vi "SaveText.vi"(7 "action":string="Save", 8 "error in":errorcluster, 10 "data in":sgl, 11 "file path (use dialog)":path) -> (0 "error out":errorcluster)   [LabVIEW 2018]
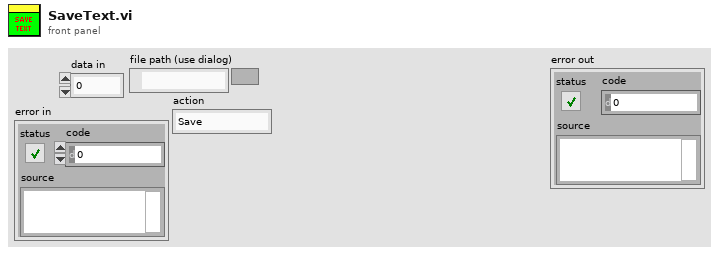
[diagram p1: front panel]
types:
  T1 = enum16{"open", "replace", "create", "open or create", "replace or create", "replace or create with confirmation"}
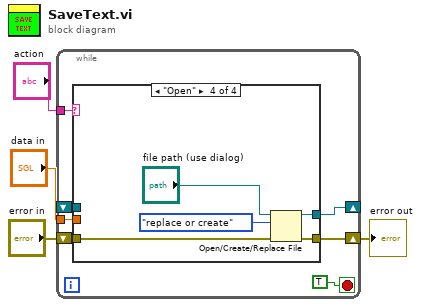
[diagram p0: block diagram]
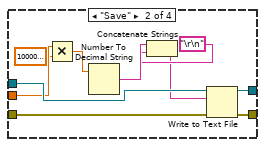
[diagram p3: hidden frame]
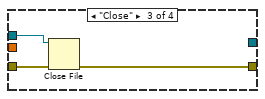
[diagram p4: hidden frame]
diagram:
  n1 = while {
    tunnel: "action" -> [w10]
    tunnel: "data in" -> [w9]
    shift-right: [w7] -> w1
    shift-left: "error in" -> [w8]
    shift-right: [w6] -> _
    shift-left: _ -> [w5]
    stop <- TRUE stop-if-true
    n2 = case shown="\"Open\"" w10 {
      tunnel: w9 -> [_ w16 _ _]
      tunnel: w8 -> [w13 w23 w26 w29]
      tunnel: [w13 w22 w24 w27] -> w7
      tunnel: [w12 w21 _ w31] -> w6
      tunnel: w5 -> [w12 w20 w25 _]
      frame "False", Default {
      }
      frame "Save" {
        n3 = Multiply(x=w16, y=sgl 1000000.0) -> (x*y=w14:sgl)
        n4 = Number To Decimal String(number=w14) -> (decimal integer string=w19:string)  [unwired: 1 in]
        n5 = Concatenate Strings(w19, "\r\n") -> (w17:string)
        n6 = Write to Text File(file (use dialog)=w20, text=w17, error in=w23) -> (refnum out=w21:refnum<file>, error out=w22:errorcluster)  [unwired: 1 in, 1 out]
      }
      frame "Close" {
        n7 = Close File(refnum=w25, error in=w26) -> (error out=w24:errorcluster)  [unwired: 1 out]
      }
      frame "Open" {
        n8 = Open/Create/Replace File(file path (use dialog)="file path (use dialog)", error in=w29, operation (0:open)=T1."replace or create") -> (refnum out=w31:refnum<file>, error out=w27:errorcluster)  [unwired: 3 in, 1 out]
      }
    }
  }
  "error out" <- w1
